vi "String_parsingV4_Single.vi"(4 "input string":string) -> (2 "V1":i32[](array[numeric]))   [LabVIEW 2014]
panel:
  out "size(s)":i32
  out "input test":u8[](array[numeric])
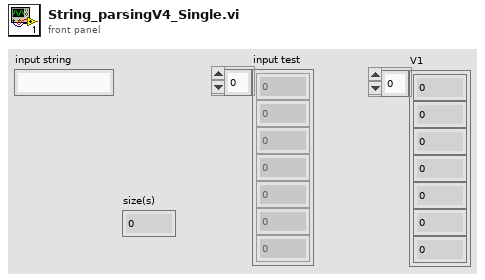
[diagram p1: front panel]
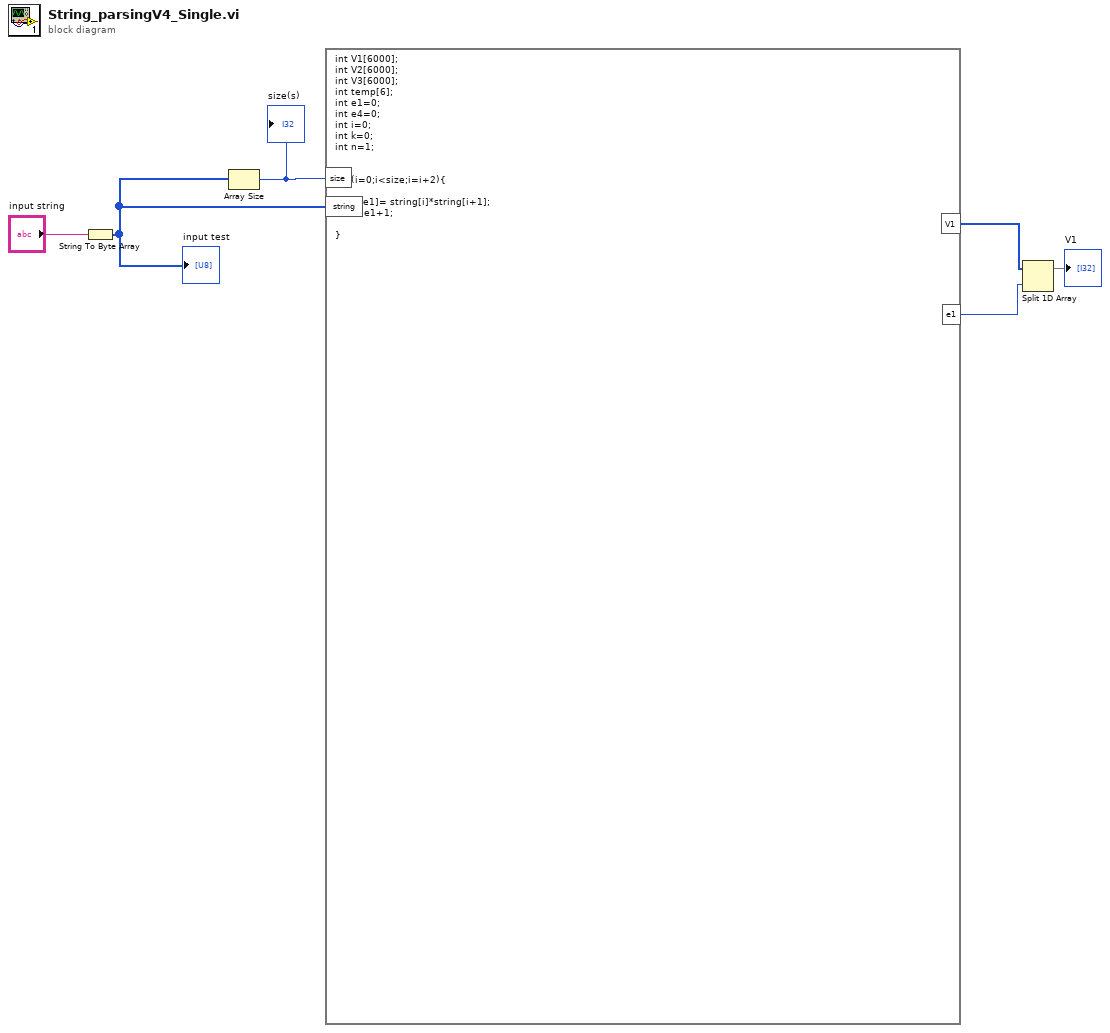
[diagram p0: block diagram]
diagram:
  n1 = String To Byte Array(string="input string") -> (unsigned byte array=w6:u8[])
  "input test" <- w6
  n2 = Array Size(array=w6) -> (size(s)=w5:i32)
  "size(s)" <- w5
  n3 = formula code="int V1[6000];\nint V2[6000];\nint V3[6000];\nint temp[6];\nint e1=0;\nint e4=0;\nint i=0;\nint k=0;\nint n=1;\n\n\nfor (i=0;i<size;i=i+2){\n \n    V1[e1]= string[i]*string[i+1];\n   e1=e1+1;\n\n}"("string"=w6, "size"=w5) -> ("V1"=w3:i32[], "e1"=w1:i32)
  n4 = Split 1D Array(array=w3, index=w1) -> (first subarray=→"V1":i32[])  [unwired: 1 out]
